vi "FF_ReadAnkleTraj.vi"(8 "error in (no error)":errorcluster, 11 "ForceField in":refnum<class "ForceField.lvclass">) -> (0 "error out":errorcluster, 2 "AnkleTraj":T1(array[cluster]), 3 "ForceField out":refnum<class "ForceField.lvclass">)   [LabVIEW 2015, in "ForceField.lvclass"]
uses:
  ForceField.lvclass
  ForceField.lvclass/ForceField.ctl
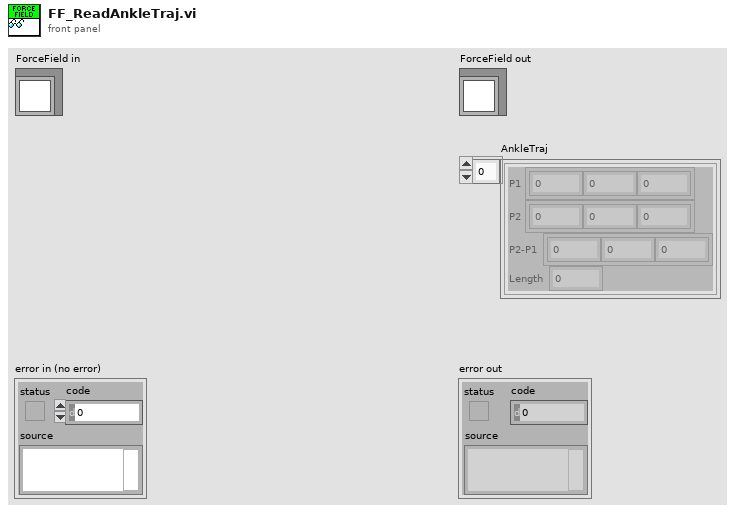
[diagram p1: front panel]
types:
  T1 = cluster{"P1":dbl[], "P2":dbl[], "P2-P1":dbl[], "Length":dbl}[]
  T2 = typedef "ForceField.lvclass/AnkleTrajPt.ctl" = cluster{"P1":dbl[], "P2":dbl[], "P1-P2":dbl[], "(P1-P2)^2":dbl}
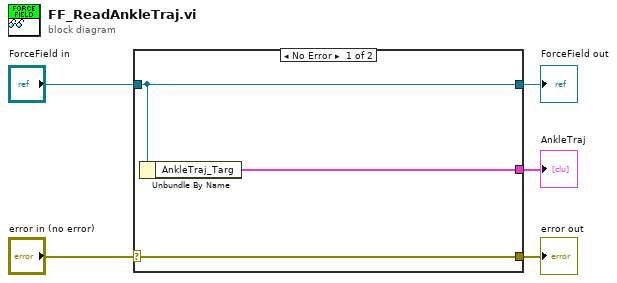
[diagram p0: block diagram]
diagram:
  n1 = case shown="No Error" "error in (no error)" {
    selector: "error in (no error)" -> [w8 w9]
    tunnel: [w8 w9] -> w4
    tunnel: [w7 w10] -> w2
    tunnel: "ForceField in" -> [w7 w10]
    tunnel: [w6 _] -> w1
    frame No Error {
      n2 = Unbundle By Name(w7) -> ("AnkleTraj_Targ"=w6:T2[])
    }
    frame Error {
    }
  }
  "error out" <- w4
  "ForceField out" <- w2
  "AnkleTraj" <- w1
